vi "RQST Lookup Table Act.vi"(7 "Action":T2, 8 "error in (no error)":errorcluster, 9 "ID":u32, 10 "Data":T3, 11 "Rqst LUT":T1) -> (0 "error out":errorcluster {"code" min=0 max=0}, 1 "Found?":bool, 2 "Data":T3, 3 "Rqst LUT out":T1)   [LabVIEW 2015, in "J1939 Addon Engine.lvlib"]
uses:
  J1939 Addon Engine.lvlib
  Types/RQST Lookup Table Reference.ctl
  Types/RQST Lookup Table Cluster.ctl
  <vilib>/xnet/xnet.llb/XNET Frame CAN.ctl
  <vilib>/xnet/xnet.llb/XNET Frame Type CAN.ctl
  Types/RQST Lookup Table Action.ctl
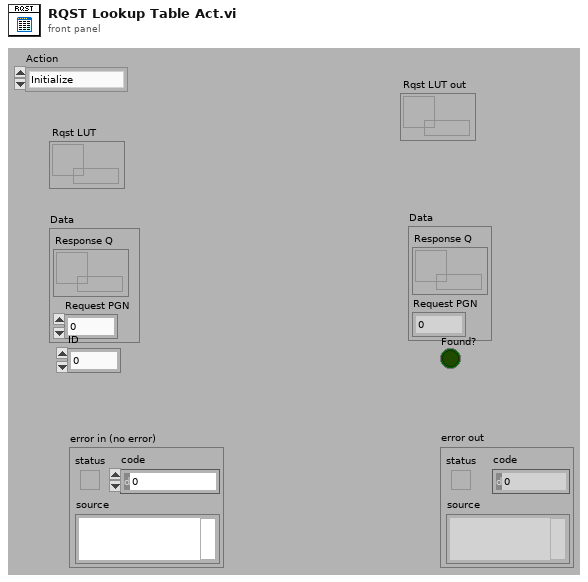
[diagram p1: front panel]
types:
  T1 = typedef "J1939 Addon Engine.lvlib/RQST Lookup Table Reference.ctl" = refnum<data-value>
  T2 = typedef "J1939 Addon Engine.lvlib/RQST Lookup Table Action.ctl" = enum16{"Initialize", "Add", "Get", "Remove"}
  T3 = typedef "J1939 Addon Engine.lvlib/RQST Lookup Table Cluster.ctl" = cluster{"Response Q":refnum<queue>, "Request PGN":u32}
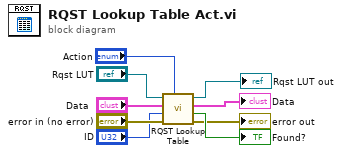
[diagram p0: block diagram]
diagram:
  n1 = call "RQST Lookup Table.vi"("Action"="Action", "error in (no error)"="error in (no error)", "ID"="ID", "Data"="Data", "Rqst LUT"="Rqst LUT") -> ("error out"=→"error out":errorcluster, "Found?"=→"Found?":bool, "Data Out"=→"Data":T3, "Rqst LUT out"=→"Rqst LUT out":T1)  [unwired: 3 in]
